vi "Write All Pages Properties.vi"(8 "error in (no error)":errorcluster, 10 "All Pages Properties":T10(array[cluster]), 11 "CustomDeviceRepo in":refnum<class "CustomDeviceRepo.lvclass">) -> (0 "error out":errorcluster, 3 "CustomDeviceRepo out":refnum<class "CustomDeviceRepo.lvclass">)   [LabVIEW 2015, in "CustomDeviceRepo.lvclass"]
uses:
  CustomDeviceRepo.lvclass
  XML Controls/Page Properties.ctl
  XML Controls/Path Cluster.ctl
  XML Controls/Help File Properties.ctl
  XML Controls/ActionVIs Properties.ctl
  XML Controls/ButtonLists Properties.ctl
  XML Controls/Button Type.ctl
  XML Controls/Dependency Properties.ctl
  XML Controls/RunTimeMenus Properties.ctl
  XML Controls/Execution Types.ctl
  CustomDeviceRepo.lvclass/CustomDeviceRepo.ctl
  VeriStand XML Parser.lvlib
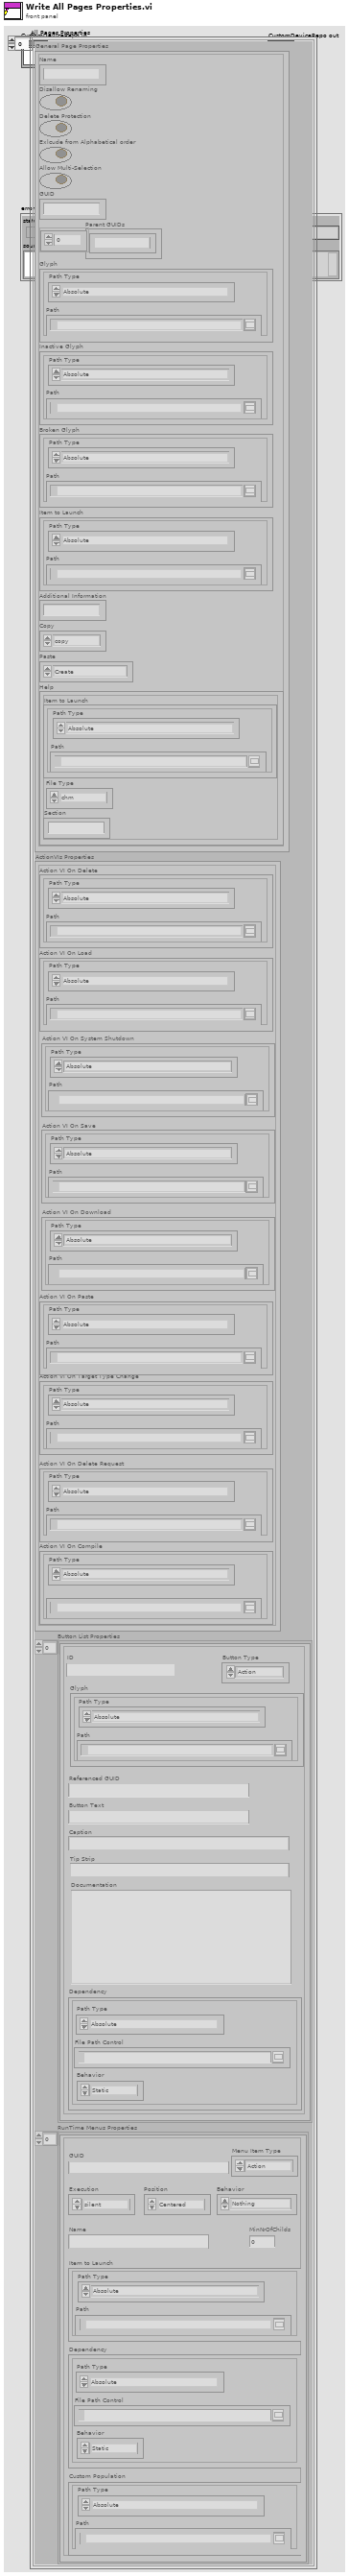
[diagram p1: front panel]
types:
  T1 = typedef "VeriStand XML Parser.lvlib/Page Properties.ctl" = cluster{"Name":string, "Disallow Renaming":bool, "Delete Protection":bool, "Exlcude from Alphabetical order":bool, "Allow Multi-Selection":bool, "GUID":string, "Parent GUIDs":string[], "Glyph":T2, "Inactive Glyph":T2, "Broken Glyph":T2, "Item to Launch":T2, "Additional Information":string, "Copy":enum16{"copy", "disabled"}, "Paste":enum16{"Create", "CreatIfNotExists_GUID", "CreatIfNotExists_Name", "Replace", "Dialog"}, "Help":T3}
  T2 = typedef "VeriStand XML Parser.lvlib/Path Cluster.ctl" = cluster{"Path":path, "Path Type":enum16{"Absolute", "To Base", "To Common Doc Dir", "To Application Data Dir"}}
  T3 = typedef "VeriStand XML Parser.lvlib/Help File Properties.ctl" = cluster{"Item to Launch":T2, "Section":string, "File Type":enum16{"chm", "other"}}
  T4 = typedef "VeriStand XML Parser.lvlib/ActionVIs Properties.ctl" = cluster{"Action VI On Delete":T2, "Action VI On Load":T2, "Action VI On Paste":T2, "Action VI On Target Type Change":T2, "Action VI On Delete Request":T2, "Action VI On Compile":T2, "Action VI On System Shutdown":T2, "Action VI On Save":T2, "Action VI On Download":T2}
  T5 = typedef "VeriStand XML Parser.lvlib/ButtonLists Properties.ctl" = cluster{"ID":string, "Glyph":T2, "Button Type":T6, "Referenced GUID":string, "Button Text":string, "Caption":string, "Tip Strip":string, "Documentation":string, "Dependency":T7}
  T6 = typedef "VeriStand XML Parser.lvlib/Button Type.ctl" = enum16{"Action", "Dialog", "Page", "Notification", "Separator"}
  T7 = typedef "VeriStand XML Parser.lvlib/Dependency Properties.ctl" = cluster{"File Path Control":path, "Path Type":enum16{"Absolute", "To Base", "To Common Doc Dir", "To Application Data Dir"}, "Behavior":enum16{"Static", "Dynamic"}}
  T8 = typedef "VeriStand XML Parser.lvlib/RunTimeMenus Properties.ctl" = cluster{"GUID":string, "Execution":T9, "MinNrOfChilds":u32, "Name":string, "Item to Launch":T2, "Dependency":T7, "Custom Population":T2, "Menu Item Type":enum16{"Action", "VI", "Separator", "Custom"}, "Behavior":enum16{"Nothing", "Open Front Panel"}, "Position":enum16{"Centered", "Mouse Pointer"}}
  T9 = typedef "VeriStand XML Parser.lvlib/Execution Types.ctl" = enum16{"silent", "modal", "floating", "default"}
  T10 = cluster{"General Page Properties":T1, "ActionVIs Properties":T4, "Button List Properties":T5[], "RunTime Menus Properties":T8[]}[]
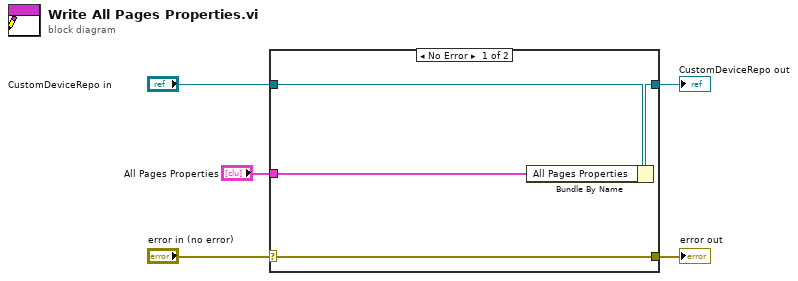
[diagram p0: block diagram]
diagram:
  n1 = case shown="No Error" "error in (no error)" {
    selector: "error in (no error)" -> [w9 w10]
    tunnel: [w9 w10] -> w4
    tunnel: [w7 w11] -> w2
    tunnel: "CustomDeviceRepo in" -> [w8 w11]
    tunnel: "All Pages Properties" -> [w6 _]
    frame No Error {
      n2 = Bundle By Name(cluster=w8, "All Pages Properties"=w6) -> (w7:refnum<class "CustomDeviceRepo.lvclass">)
    }
    frame Error {
    }
  }
  "error out" <- w4
  "CustomDeviceRepo out" <- w2
